vi "Close Project.vi"(8 "error in":errorcluster, 10 "save":bool=TRUE, 11 "project ref":refnum<vi>) -> (0 "error out":errorcluster)   [LabVIEW 2024, in "gRPC Client Generation.lvlib"]
uses:
  gRPC Client Generation.lvlib
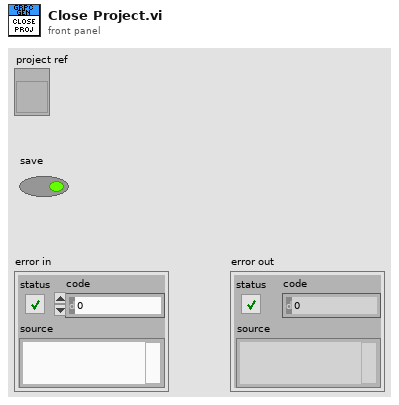
[diagram p1: front panel]
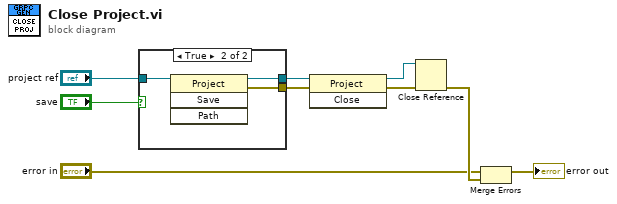
[diagram p0: block diagram]
diagram:
  n1 = case shown="True" "save" {
    tunnel: "project ref" -> [w10 w13]
    tunnel: [w10 w12] -> w7
    tunnel: [_ w11] -> w6
    frame False {
    }
    frame True {
      n2 = invoke class="Project" method="Save"(reference=w13) -> (reference out=w12:refnum<vi>, error out=w11:errorcluster)  [unwired: 3 in, 2 out]
    }
  }
  n3 = invoke class="Project" method="Close"(reference=w7, error in=w6) -> (reference out=w4:refnum<vi>, error out=w5:errorcluster)  [unwired: 1 in, 1 out]
  n4 = Close Reference(reference=w4, error in (no error)=w5) -> (error out=w3:errorcluster)
  n5 = Merge Errors("error in", w3) -> (→"error out":errorcluster)
